vi "SetVelocity.vi"(8 "error in":errorcluster, 9 "Velocity":dbl, 11 "VISA resource":refnum<visa-resource-name>) -> (0 "error out":errorcluster)   [LabVIEW 2012, in "Micos_uic.lvlib"]
uses:
  <instrlib>/Micos_uic/Micos_uic.lvlib
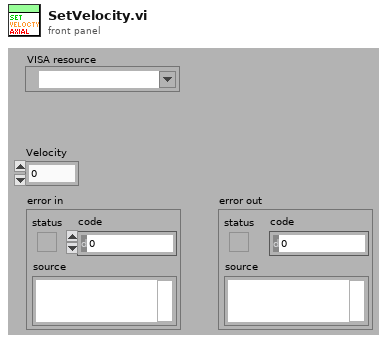
[diagram p1: front panel]
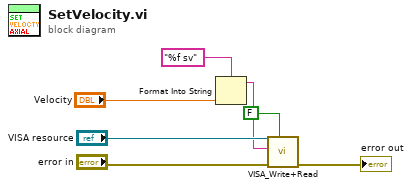
[diagram p0: block diagram]
diagram:
  n1 = Format Into String(format string="%f sv", "Velocity") -> (resulting string=w3:string)  [unwired: 2 in, 1 out]
  n2 = call <instrlib>:"VISA_Write+Read.vi"("Read?"=FALSE, "error in (no error)"="error in", "Write Buffer"=w3, "VISA resource name"="VISA resource") -> ("error out"=→"error out":errorcluster)  [unwired: 5 in, 2 out]
